vi "dfd_Calculate Output Iwl.vi"(9 "sum iwl":i16, 10 "gain value":dbl, 11 "gain wl":i16) -> (3 "output iwl":i16)   [LabVIEW 2017, in "NI_DigFilter_FXP.lvlib"]
uses:
  <vilib>/addons/Digital Filter Design/NI_DigFilter_FXP.lvlib
  <vilib>/addons/Digital Filter Design/NI_DigFilterLicensed.lvlib
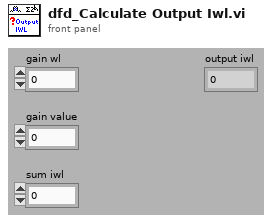
[diagram p1: front panel]
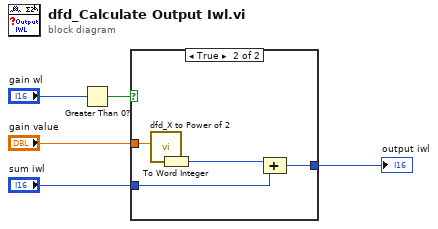
[diagram p0: block diagram]
diagram:
  n1 = Greater Than 0?(x="gain wl") -> (x > 0?=w1:bool)
  n2 = case shown="True" w1 {
    tunnel: [w6 w11] -> w5
    tunnel: "sum iwl" -> [w6 w10]
    tunnel: "gain value" -> [_ w8]
    frame False {
    }
    frame True {
      n3 = call <vilib>:"dfd_X to Power of 2.vi"("x"=w8) -> ("n"=w9:dbl)  [unwired: 10 out]
      n4 = To Word Integer(number=w9) -> (16bit integer=w7:i16)
      n5 = Compound Arithmetic op=ADD(w7, w10) -> (w11:i16)
    }
  }
  "output iwl" <- w5
